vi "lectura_de_datos_!.vi"() -> ()   [LabVIEW 2020]
panel:
  out "Waveform Graph":dynamicdata(graph)
  in  "stop":bool
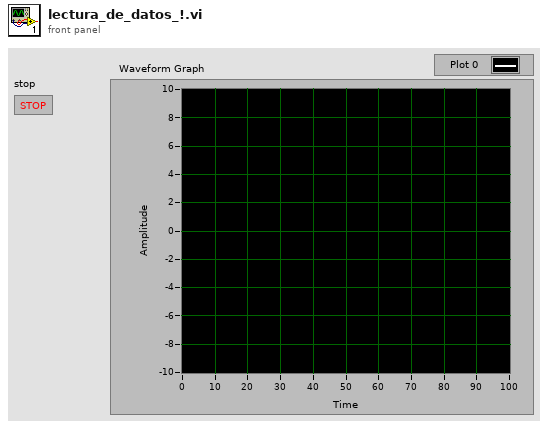
[diagram p1: front panel]
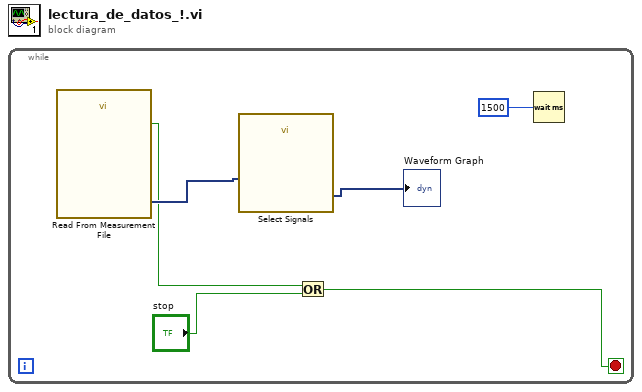
[diagram p0: block diagram]
diagram:
  n1 = while {
    stop <- w2 stop-if-true
    n2 = call "Read From Measurement File"() -> ("Signals"=w6:dynamicdata, "EOF?"=w4:bool)  [unwired: 6 in, 4 out]
    n3 = call "Select Signals"("Signals"=w6) -> ("Signal Out"=→"Waveform Graph":dynamicdata)  [unwired: 9 in, 1 out]
    n4 = Or(x=w4, y="stop") -> (x .or. y?=w2:bool)
    n5 = Wait (ms)(milliseconds to wait=u32 1500 ("millisecond timer value")) -> ()  [unwired: 1 out]
  }
